vi "get_index_and_value_from_key.vi"(8 "error in (no error)":errorcluster, 10 "key":string, 11 "Map.lvclass in":refnum<class "Map.lvclass">) -> (0 "error out":errorcluster, 1 "submap":refnum<class "Map.lvclass">, 2 "value":variant, 3 "Map.lvclass out":refnum<class "Map.lvclass">, 4 "submap?":bool, 5 "key exists?":bool, 6 "index":i32)   [LabVIEW 2010, in "Map.lvclass"]
doc: "This method returns a direct entry of a map (you can't access entries further down the hierarchy in the case of a nested map), plus its index in the internal array.\nIf the value is a Map itself, it is tconverted to a Map, returned as \"submap\" and \"submap?\" is true.\nIf the key given is not found, \"key exists?\" is false, and \"index\" is -1."
uses:
  Map.lvclass
  Map.lvclass/Map.ctl
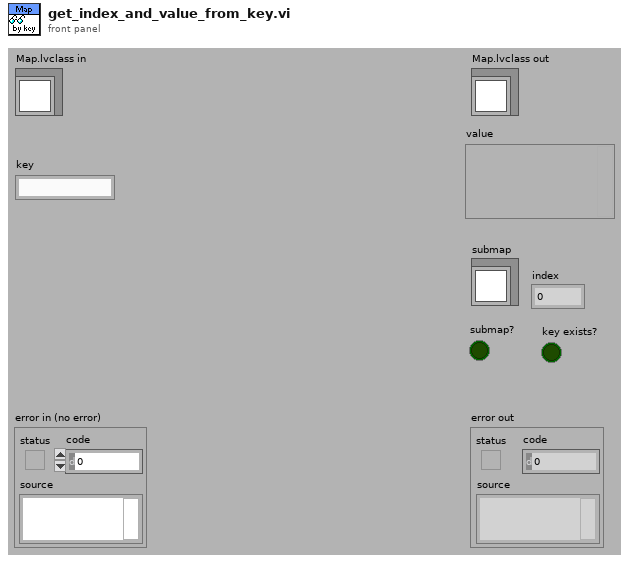
[diagram p1: front panel]
types:
  T1 = typedef "Map.lvclass/element_cluster.ctl" = cluster{"key":string, "value":variant}
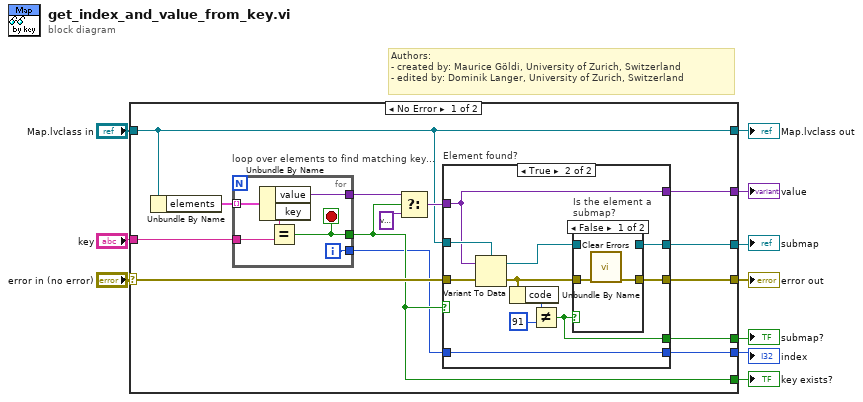
[diagram p0: block diagram]
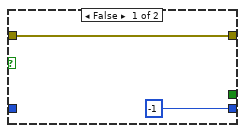
[diagram p2: hidden frame]
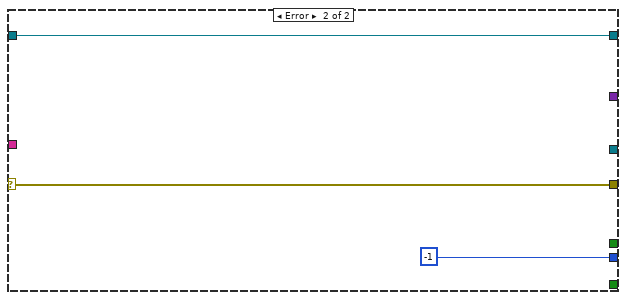
[diagram p4: hidden frame]
diagram:
  # "Authors: \n- created by: Maurice Göldi, University of Zurich, Switzerland\n- edited by: Dominik Langer, University of Zurich, Switzerland"
  n1 = case shown="No Error" "error in (no error)" {
    selector: "error in (no error)" -> [w16 w49]
    tunnel: [w24 w49] -> w9
    tunnel: [w11 w50] -> w8
    tunnel: "Map.lvclass in" -> [w11 w50]
    tunnel: [w22 _] -> w7
    tunnel: [w21 _] -> w6
    tunnel: [w23 _] -> w5
    tunnel: [w15 _] -> w3
    tunnel: [w20 -1] -> w2
    tunnel: "key" -> [w13 _]
    frame No Error {
      n2 = Unbundle By Name(w11) -> ("elements"=w17:T1[])
      n3 = for "loop over elements to find matching key..." {
        tunnel: w17 -> [w30] mode=indexing
        tunnel: w13 -> [w28]
        tunnel: [w27] -> w15
        tunnel: [w26] -> w12
        tunnel: [w25] -> w19
        i -> [w26]
        stop <- w27 stop-if-true
        n4 = Unbundle By Name(w30) -> ("value"=w25:variant, "key"=w29:string)
        n5 = Equal?(x=w29, y=w28) -> (x = y?=w27:bool)
      }
      n6 = Select(t=w19, s=w15, f=variant ("value")) -> (s? t:f=w14:variant)
      n7 = case "Element found?" shown="True" w15 {
        tunnel: w16 -> [w32 w43]
        tunnel: [w32 w42] -> w24
        tunnel: [_ w33] -> w22
        tunnel: w11 -> [_ w41]
        tunnel: [_ w35] -> w23
        tunnel: [_ w36] -> w21
        tunnel: [-1 w34] -> w20
        tunnel: w12 -> [_ w34]
        tunnel: w14 -> [_ w33]
        frame False {
        }
        frame True {
          n8 = Variant To Data(error in=w43, Variant=w33, type=w41) -> (error out=w40:errorcluster, data=w37:refnum<class "Map.lvclass">)
          n9 = Unbundle By Name(w40) -> ("code"=w38:i32)
          n10 = Not Equal?(x=w38, y=91 ("x")) -> (x != y?=w35:bool)
          n11 = case "Is the element a submap?" shown="False" w35 {
            tunnel: w40 -> [w45 w47]
            tunnel: [w44 w47] -> w42
            tunnel: w37 -> [_ w46]
            tunnel: [_ w46] -> w36
            frame False {
              n12 = call <vilib>:"Clear Errors.vi"("error in (no error)"=w45) -> ("error out"=w44:errorcluster)  [unwired: 6 out]
            }
            frame True {
            }
          }
        }
      }
    }
    frame Error {
    }
  }
  "error out" <- w9
  "Map.lvclass out" <- w8
  "submap?" <- w5
  "value" <- w7
  "submap" <- w6
  "key exists?" <- w3
  "index" <- w2
